vi "writeExpInfo.vi"() -> ()   [LabVIEW 2014, in "ChirpV2.lvclass"]
uses:
  EIS/Electrochemical Instrument Folder/Chirp_OOP/ChirpV2.lvclass
  <vilib>/addons/database/Connection.llb/DB Tools Open Connec (String).vi
  <vilib>/addons/database/NI_Database_API.lvlib
panel:
  out "error out":errorcluster
  in  "Exp_Info":T1 {"Time Stamp" format="%<%H:%M:%S\n%Y/%m/%d>T"}
  in  "db_File":path=path "C:/Users/YuanYuan/Desktop/Labview Data/Database"
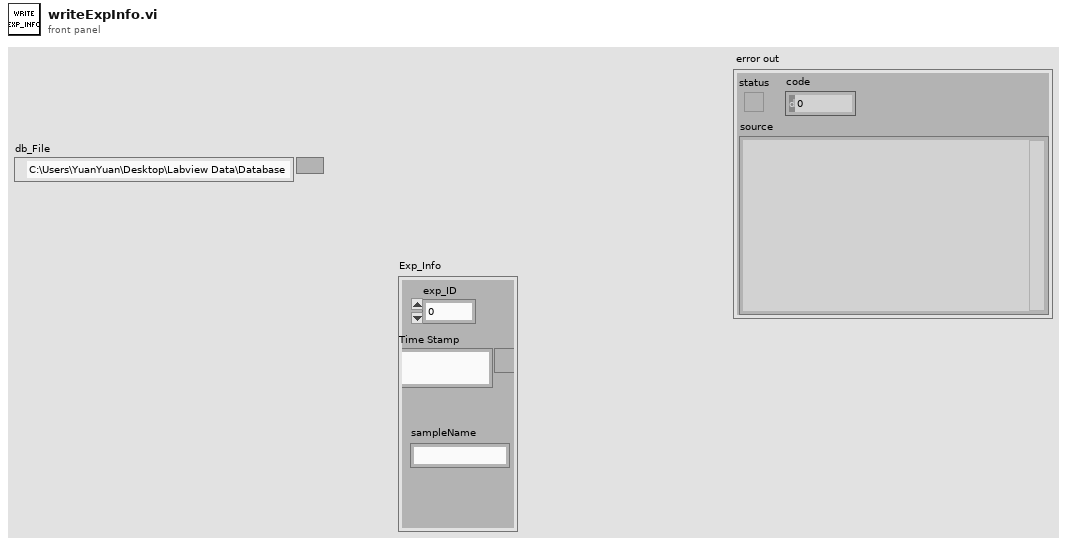
[diagram p1: front panel]
types:
  T1 = cluster{"exp_ID":i32, "Time Stamp":timestamp, "sampleName":string}
  T2 = typedef "NI_Database_API.lvlib/Conn ObjectReference.ctl" = refnum<k1>
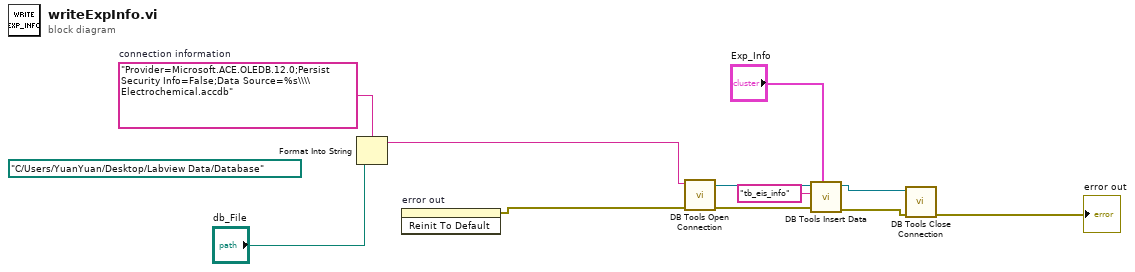
[diagram p0: block diagram]
diagram:
  (unwired) path "C:/Users/YuanYuan/Desktop/Labview Data/Database" ("path")
  w11 = "Provider=Microsoft.ACE.OLEDB.12.0;Persist Security Info=False;Data Source=%s\\\\Electrochemical.accdb"  # connection information
  n1 = Format Into String(format string=w11, "db_File") -> (resulting string=w9:string)  [unwired: 2 in, 1 out]
  n2 = invoke on="error out" class="Clust (strict)" method="Reinit To Default"() -> (error out=w1:errorcluster)  [unwired: 3 in, 2 out]
  n3 = call-poly <vilib>:"DB Tools Open Connection.vi"("error in (no error)"=w1, "connection information"=w9) -> ("error out"=w7:errorcluster, "connection reference"=w8:T2)  [unwired: 6 in]
  n4 = call <vilib>:"DB Tools Insert Data.vi"("data"="Exp_Info", "error in (no error)"=w7, "table"="tb_eis_info", "connection reference"=w8) -> ("error out"=w2:errorcluster, "connection reference out"=w3:T2)  [unwired: 6 in]
  n5 = call <vilib>:"DB Tools Close Connection.vi"("error in (no error)"=w2, "connection reference"=w3) -> ("error out"=→"error out":errorcluster)  [unwired: 5 in]
